vi "elapsed_sec_to_timestamp.vi"(11 "Input Elapsed Seconds":dbl=86397.0) -> (3 "Timestamp":string="23:59:57")   [LabVIEW 2021]
panel:
  out "Sec":dbl=57.00000000000273
  out "Hr":dbl=23.0
  out "Min":dbl=59.00000000000006
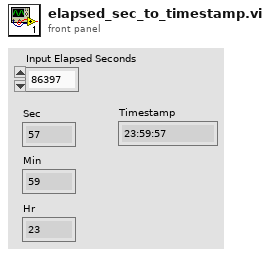
[diagram p1: front panel]
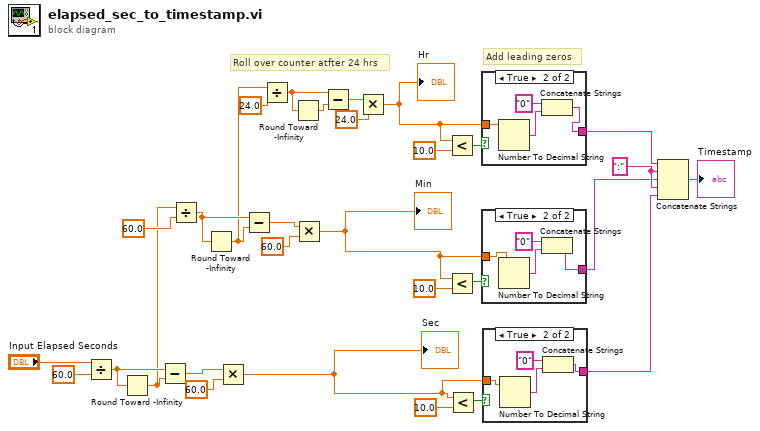
[diagram p0: block diagram]
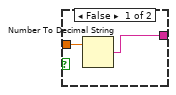
[diagram p2: hidden frame]
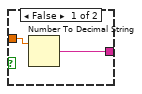
[diagram p3: hidden frame]
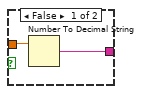
[diagram p4: hidden frame]
diagram:
  w30 = ":" ("string")
  # "Roll over counter atfter 24 hrs"
  # "Add leading zeros"
  n1 = Divide(x="Input Elapsed Seconds", y=60.0) -> (x/y=w25:dbl)
  n2 = Round Toward -Infinity(1:w25) -> (0:w19:dbl)
  n3 = Subtract(x=w25, y=w19) -> (x-y=w27:dbl)
  n4 = Divide(x=w19, y=60.0) -> (x/y=w23:dbl)
  n5 = Round Toward -Infinity(1:w23) -> (0:w6:dbl)
  n6 = Multiply(x=w27, y=60.0) -> (x*y=w10:dbl)
  "Sec" <- w10
  n7 = Subtract(x=w23, y=w6) -> (x-y=w21:dbl)
  n8 = Divide(x=w6, y=24.0) -> (x/y=w4:dbl)
  n9 = Round Toward -Infinity(1:w4) -> (0:w5:dbl)
  n10 = Multiply(x=w21, y=60.0) -> (x*y=w13:dbl)
  "Min" <- w13
  n11 = Subtract(x=w4, y=w5) -> (x-y=w3:dbl)
  n12 = Multiply(x=w3, y=24.0) -> (x*y=w1:dbl)
  "Hr" <- w1
  n13 = Less?(x=w1, y=10.0) -> (x < y?=w15:bool)
  n14 = Less?(x=w13, y=10.0) -> (x < y?=w11:bool)
  n15 = Less?(x=w10, y=10.0) -> (x < y?=w9:bool)
  n16 = case shown="True" w15 {
    tunnel: w1 -> [w32 w34]
    tunnel: [w31 w33] -> w14
    frame False {
      n17 = Number To Decimal String(number=w32) -> (decimal integer string=w31:string)  [unwired: 1 in]
    }
    frame True {
      n18 = Number To Decimal String(number=w34) -> (decimal integer string=w36:string)  [unwired: 1 in]
      n19 = Concatenate Strings("0" ("string"), w36) -> (w33:string)
    }
  }
  n20 = case shown="True" w11 {
    tunnel: w13 -> [w38 w40]
    tunnel: [w37 w39] -> w12
    frame False {
      n21 = Number To Decimal String(number=w38) -> (decimal integer string=w37:string)  [unwired: 1 in]
    }
    frame True {
      n22 = Number To Decimal String(number=w40) -> (decimal integer string=w42:string)  [unwired: 1 in]
      n23 = Concatenate Strings("0" ("string"), w42) -> (w39:string)
    }
  }
  n24 = case shown="True" w9 {
    tunnel: w10 -> [w44 w45]
    tunnel: [w43 w46] -> w8
    frame False {
      n25 = Number To Decimal String(number=w44) -> (decimal integer string=w43:string)  [unwired: 1 in]
    }
    frame True {
      n26 = Number To Decimal String(number=w45) -> (decimal integer string=w48:string)  [unwired: 1 in]
      n27 = Concatenate Strings("0" ("string"), w48) -> (w46:string)
    }
  }
  n28 = Concatenate Strings(w14, w30, w12, w30, w8) -> (→"Timestamp":string)
